vi "Check Sudoku Formal by Int.vi"(8 "error in (no error)":errorcluster, 11 "Sudoku Class in":refnum<class "Sudoku Class.lvclass">) -> (0 "error out":errorcluster, 1 "Is Modify":bool, 2 "Sudoku Formal Out":T1, 3 "Sudoku Class out":refnum<class "Sudoku Class.lvclass">)   [LabVIEW 2015, in "Sudoku Library.lvlib" / "Sudoku Class.lvclass"]
doc: "Created IvanLis by LabVIEW Portal\nProfile: http://labviewportal.org/memberlist.php?mode=viewprofile&u=987\neMail: IvanLisanov@gMail.com\nTelegram: https://t.me/IvanLis"
uses:
  Sudoku Class.lvclass
  TypeDef/Sudoku Formal.ctl
  TypeDef/Cell Formal.ctl
  Sudoku Class.lvclass/Sudoku Class.ctl
  Sudoku Library.lvlib
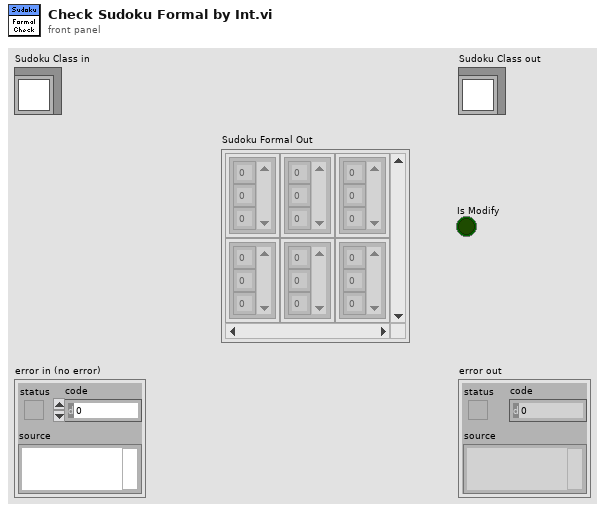
[diagram p1: front panel]
types:
  T1 = typedef "Sudoku Library.lvlib/Sudoku Formal.ctl" = T2[][]
  T2 = typedef "Sudoku Library.lvlib/Cell Formal.ctl" = cluster{"Variant":u8[]}
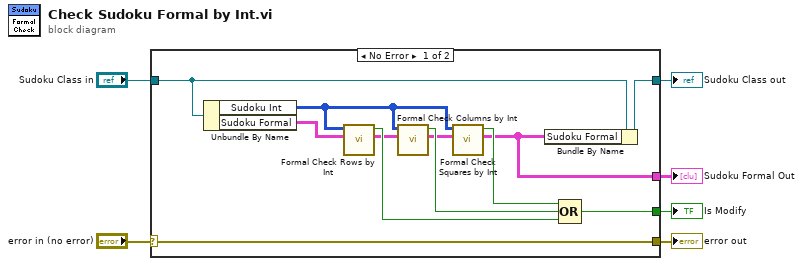
[diagram p0: block diagram]
diagram:
  n1 = case shown="No Error" "error in (no error)" {
    selector: "error in (no error)" -> [w18 w20]
    tunnel: [w18 w20] -> w5
    tunnel: [w16 w19] -> w3
    tunnel: "Sudoku Class in" -> [w17 w19]
    tunnel: [w11 _] -> w2
    tunnel: [w8 _] -> w1
    frame No Error {
      n2 = Unbundle By Name(w17) -> ("Sudoku Int"=w7:u8[][], "Sudoku Formal"=w15:T1)
      n3 = call "Formal Check Rows by Int.vi"("Sudoku Formal In"=w15, "Sudoku Int"=w7) -> ("Sudoku Formal Out"=w10:T1, "Is Modify"=w12:bool)  [unwired: 8 in]
      n4 = call "Formal Check Columns by Int.vi"("Sudoku Formal In"=w10, "Sudoku Int"=w7) -> ("Sudoku Formal Out"=w9:T1, "Is Modify"=w13:bool)  [unwired: 8 in]
      n5 = call "Formal Check Squares by Int.vi"("Sudoku Formal In"=w9, "Sudoku Int"=w7) -> ("Sudoku Formal Out"=w8:T1, "Is Modify"=w14:bool)  [unwired: 8 in]
      n6 = Bundle By Name(cluster=w17, "Sudoku Formal"=w8) -> (w16:refnum<class "Sudoku Class.lvclass">)
      n7 = Compound Arithmetic op=OR(w14, w13, w12) -> (w11:bool)
    }
    frame Error {
    }
  }
  "error out" <- w5
  "Sudoku Class out" <- w3
  "Is Modify" <- w2
  "Sudoku Formal Out" <- w1
